vi "Save-Recall Setup.vi"(8 "error in (no error)":errorcluster, 9 "Memory Address (0)":i32, 10 "Action (0: Save)":i32(ring) items=["Save", "Recall"], 11 "VISA resource name":refnum<visa-resource-name>) -> (0 "error out":errorcluster, 3 "VISA resource name out":refnum<visa-resource-name>)   [LabVIEW 2012, in "Tektronix TDS 200 1000 2000 Series.lvlib"]
doc: "Saves and recalls oscilloscope settings from internal memory."
uses:
  <instrlib>/Tektronix TDS 200 1000 2000 Series/Tektronix TDS 200 1000 2000 Series.lvlib
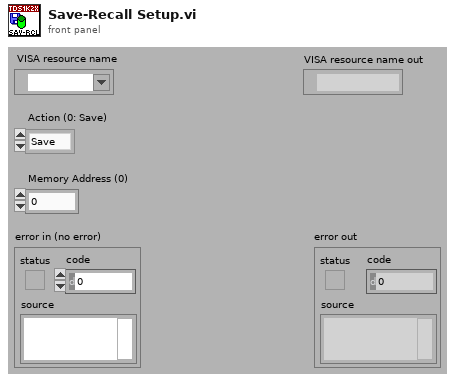
[diagram p1: front panel]
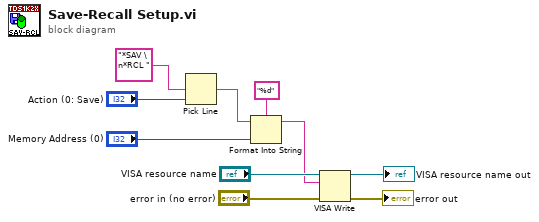
[diagram p0: block diagram]
diagram:
  n1 = Pick Line(multi-line string="*SAV \n*RCL " ("initial string"), line index="Action (0: Save)") -> (output string=w7:string)  [unwired: 1 out]
  n2 = Format Into String(format string="%d", initial string=w7, "Memory Address (0)") -> (resulting string=w2:string)  [unwired: 1 in, 1 out]
  n3 = VISA Write(VISA resource name="VISA resource name", write buffer=w2, error in (no error)="error in (no error)") -> (VISA resource name out=→"VISA resource name out":refnum<visa-resource-name>, error out=→"error out":errorcluster)  [unwired: 1 out]
